vi "_Main_04_look_only.vi"() -> ()   [LabVIEW 2017]
panel:
  out "Red LED":bool
  out "Ramping":bool
  out "Heater\nEnabled":bool
  out "Heating":bool
  out "Green LED":bool
  out "unsigned 16bit integer":u16
  in  "Speed, K/min":dbl=5.0 min=0.1 max=10.0
  in  "Target, K":dbl=295.0 min=195.0 max=395.0
  in  "Ramp":bool
  out "Power LOG":cluster{dbl[], dbl[]}(graph)
  in  "Set temp":dbl=195.0 min=195.0 max=395.0
  in  "Setpoint":bool
  out "TrigTimer, s":dbl
  out "Vout, V":dbl format="%#.2g"
  out "Vin, V":dbl format="%#.5g"
  out "Temp, K":dbl
  out "Temp_sp, K":dbl
  out "Temp_gsp, K":dbl
  out "Temp LOG":cluster{dbl[], dbl[]}(graph)
  out "Bytes at Port":u32
  out "RecTry":i32
  in  "Stop Button":bool
  in  "COM port":refnum<visa-resource-name>
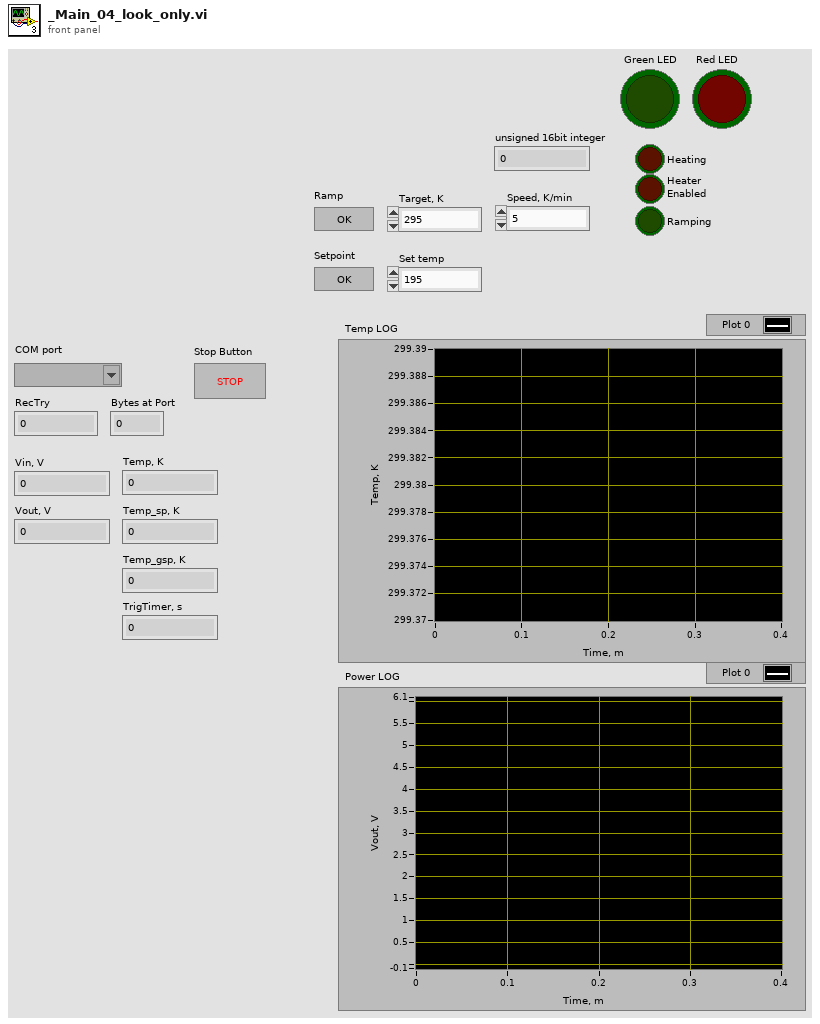
[diagram p1: front panel]
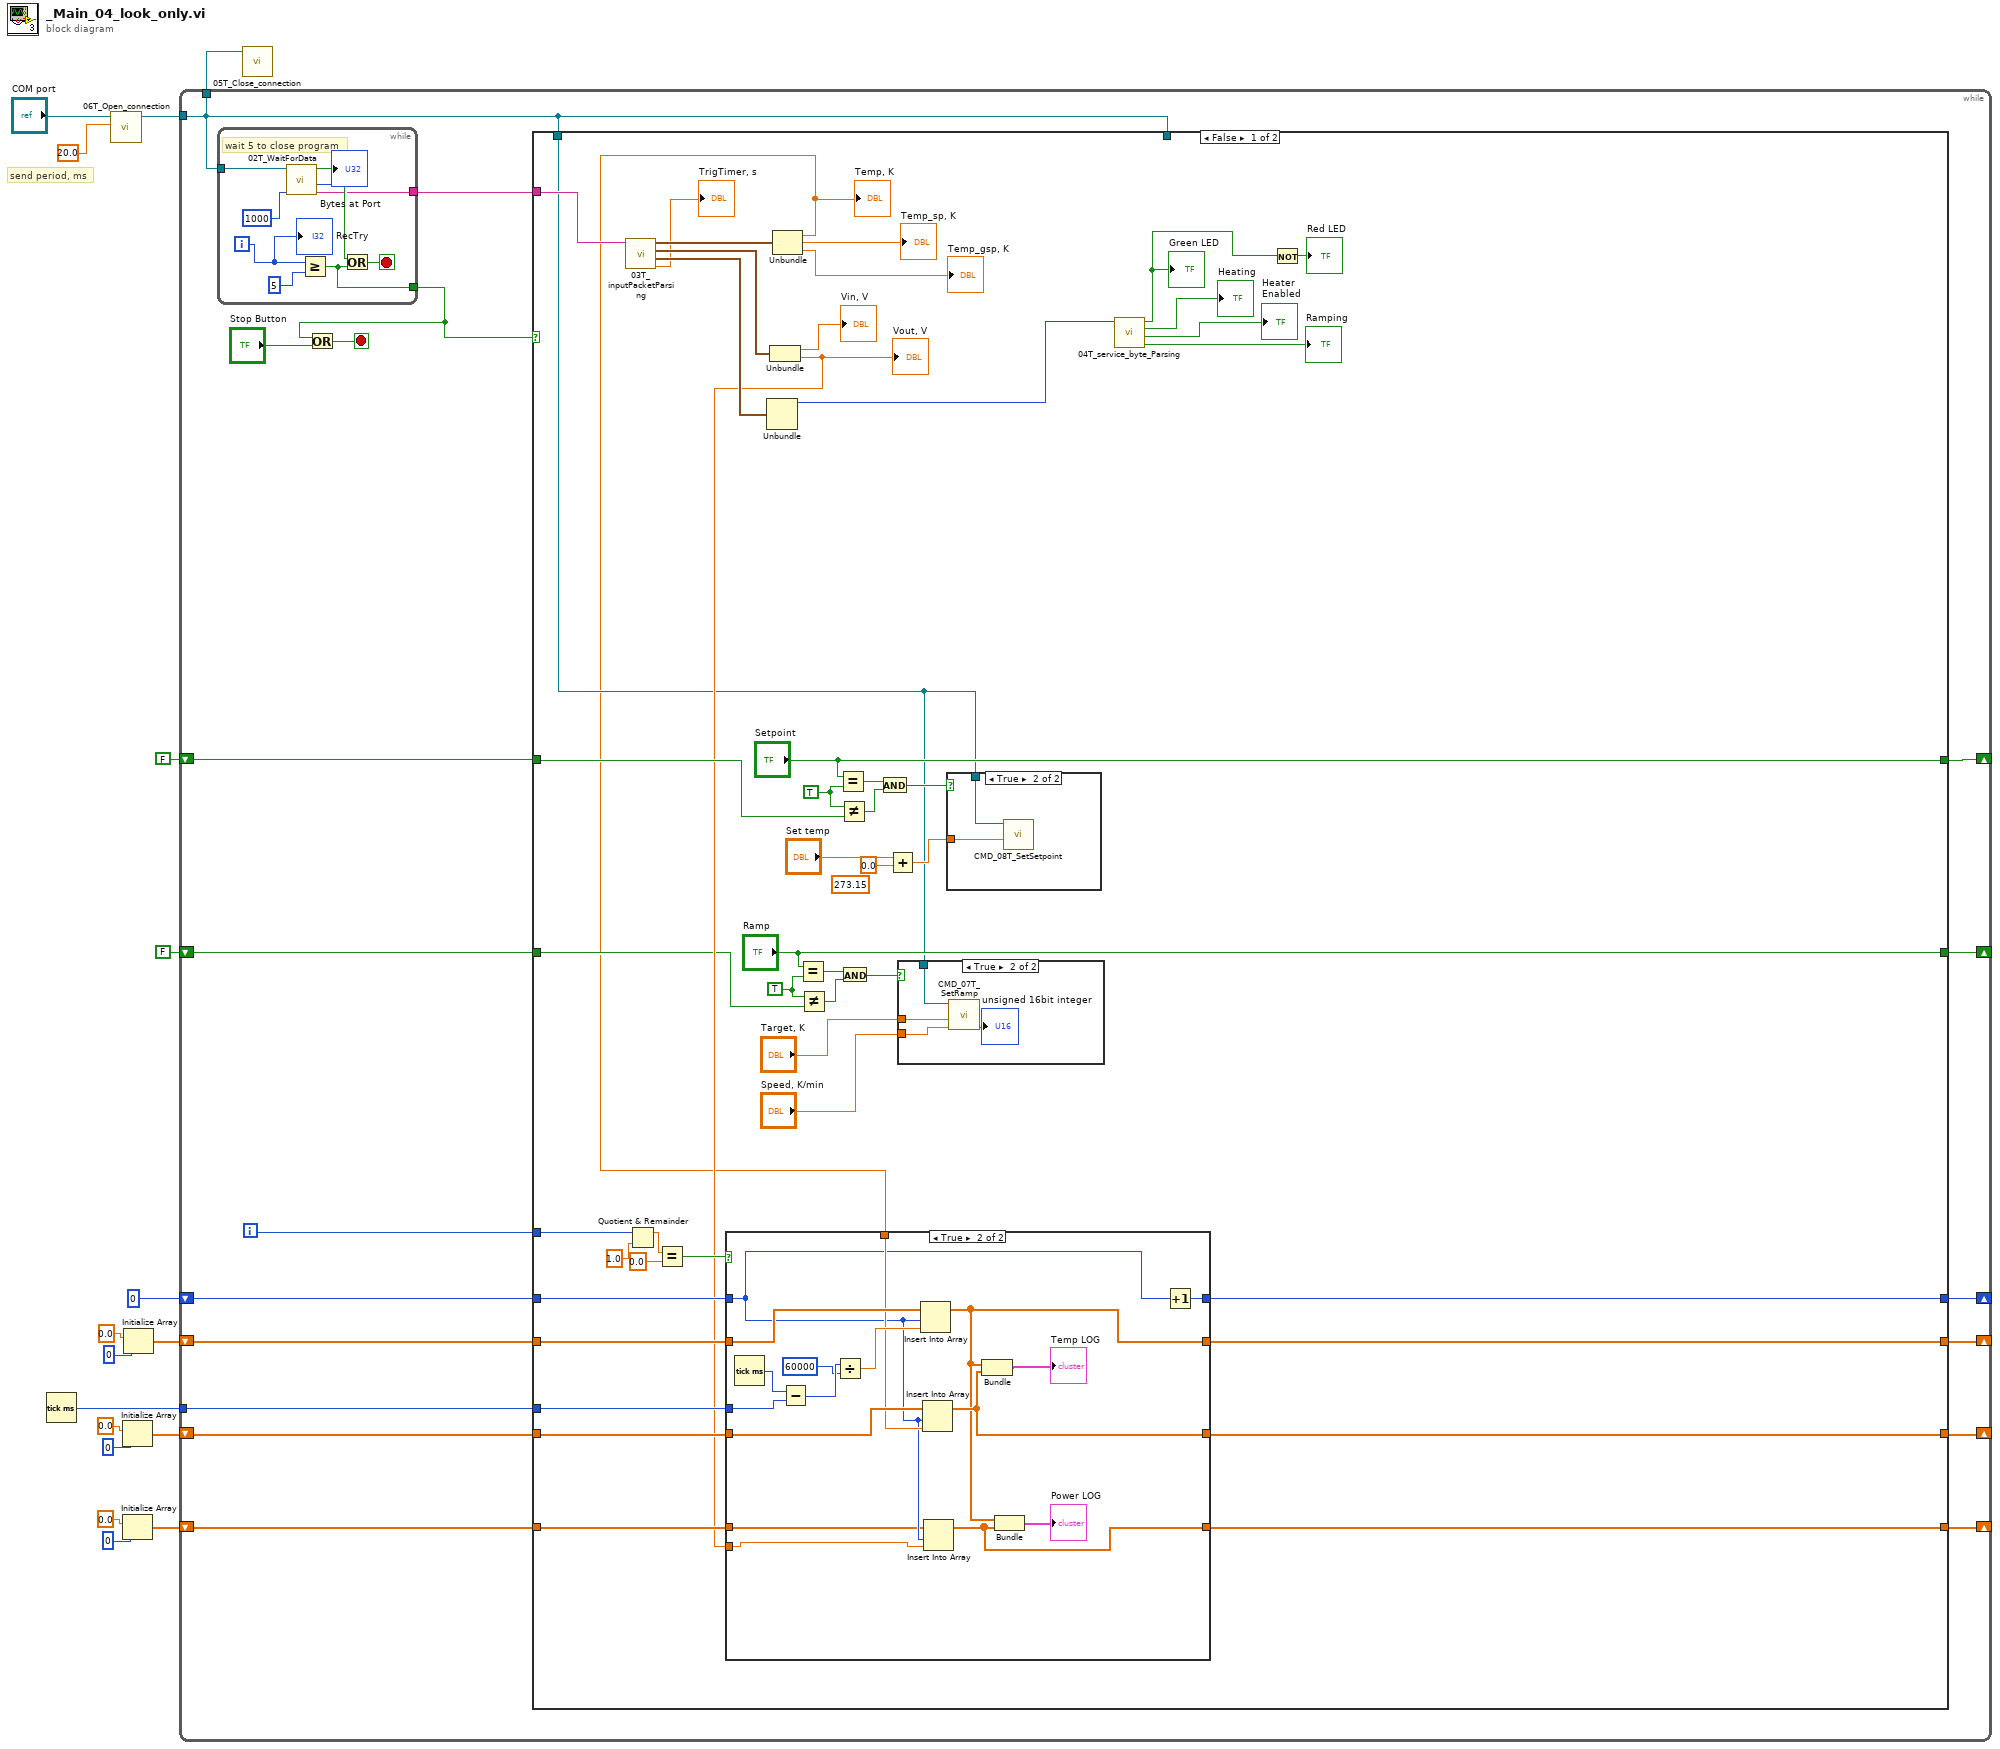
[diagram p0: block diagram]
diagram:
  # "send period, ms"
  n1 = Tick Count (ms)() -> (millisecond timer value=w13:u32)
  n2 = call "06T_Open_connection.vi"("Period, ms"=20.0, "COM port"="COM port") -> ("VISA"=w3:refnum<visa-resource-name>)  [unwired: 9 in]
  n3 = Initialize Array(0.0 ("element"), 0 ("dimension size")) -> (w10:dbl[])
  n4 = Initialize Array(0.0 ("element"), 0 ("dimension size")) -> (w6:dbl[])
  n5 = Initialize Array(0.0 ("element"), 0 ("dimension size")) -> (w14:dbl[])
  n6 = while {
    tunnel: w3 -> [w22]
    tunnel: [w22] -> w4
    shift-right: [w31] -> _
    shift-left: 0 -> [w32]
    tunnel: w13 -> [w29]
    shift-right: [w27] -> _
    shift-left: w14 -> [w30]
    shift-right: [w26] -> _
    shift-left: w10 -> [w28]
    shift-right: [w24] -> _
    shift-left: FALSE ("OK Button") -> [w23]
    shift-right: [w20] -> _
    shift-left: w6 -> [w21]
    shift-right: [w19] -> _
    shift-left: FALSE ("Ramp") -> [w18]
    i -> [w33]
    stop <- w36 stop-if-true
    n7 = while {
      tunnel: w22 -> [w118]
      tunnel: [w121] -> w35
      tunnel: [w122] -> w34
      i -> [w120]
      stop <- w124 stop-if-true
      # "wait 5 to close program"
      n8 = call "02T_WaitForData.vi"("WaitTimeoutMS"=u32 1000, "VISA"=w118) -> ("Buffer"=w122:string, "Bytes at Port"=→"Bytes at Port":u32, "Data Recived"=w123:bool)  [unwired: 7 in]
      n9 = Greater Or Equal?(x=w120, y=5) -> (x >= y?=w121:bool)
      n10 = Or(x=w123, y=w121) -> (x .or. y?=w124:bool)
      "RecTry" <- w120
    }
    n11 = Or(x=w35, y="Stop Button") -> (x .or. y?=w36:bool)
    n12 = case shown="False" w35 {
      tunnel: w34 -> [w75 _]
      tunnel: w33 -> [w81 _]
      tunnel: w22 -> [_ _]
      tunnel: w32 -> [w79 w117]
      tunnel: [w78 w117] -> w31
      tunnel: w30 -> [w68 w116]
      tunnel: w29 -> [w77 _]
      tunnel: w28 -> [w66 w115]
      tunnel: [w76 w116] -> w27
      tunnel: [w59 w115] -> w26
      tunnel: ["Setpoint" w114] -> w24
      tunnel: w23 -> [w63 w114]
      tunnel: w22 -> [w46 _]
      tunnel: w21 -> [w55 w113]
      tunnel: [w54 w113] -> w20
      tunnel: ["Ramp" w112] -> w19
      tunnel: w18 -> [w48 w112]
      frame False {
        w49 = TRUE ("y")
        (unwired) 273.15 ("y")
        w62 = TRUE ("x")
        n13 = call "03T_inputPacketParsing.vi"("string"=w75) -> ("TrigTimer, s"=→"TrigTimer, s":dbl, "Service"=w70:cluster{i32, i32, i32, i32}, "Voltage"=w71:cluster{dbl, dbl}, "Temp"=w74:cluster{dbl, dbl, dbl})  [unwired: 7 in]
        n14 = Quotient & Remainder(x=w81, y=1.0) -> (x-y*floor(x/y)=w84:dbl)  [unwired: 1 out]
        n15 = Equal?(x=w84, y=0.0) -> (x = y?=w80:bool)
        n16 = Unbundle(w70) -> (w43:i32)  [unwired: 3 out]
        n17 = Unbundle(w71) -> (→"Vin, V":dbl, w53:dbl)
        "Vout, V" <- w53
        n18 = Unbundle(w74) -> (w39:dbl, →"Temp_sp, K":dbl, →"Temp_gsp, K":dbl)
        "Temp, K" <- w39
        n19 = case shown="True" w80 {
          tunnel: w79 -> [w94 w100]
          tunnel: [w94 w107] -> w78
          tunnel: w68 -> [w92 w105]
          tunnel: w77 -> [_ w110]
          tunnel: w66 -> [w93 w104]
          tunnel: [w93 w102] -> w59
          tunnel: [w92 w98] -> w76
          tunnel: w39 -> [_ w101]
          tunnel: w55 -> [w91 w99]
          tunnel: [w91 w96] -> w54
          tunnel: w53 -> [_ w95]
          frame False {
          }
          frame True {
            n20 = Tick Count (ms)() -> (millisecond timer value=w111:u32)
            n21 = Subtract(x=w111, y=w110) -> (x-y=w109:u32)
            n22 = Divide(x=w109, y=u32 60000) -> (x/y=w106:dbl)
            n23 = Insert Into Array(array=w105, index=w100, new element=w106) -> (w98:dbl[])
            n24 = Insert Into Array(array=w104, index=w100, new element=w101) -> (w102:dbl[])
            n25 = Insert Into Array(array=w99, index=w100, new element=w95) -> (w96:dbl[])
            n26 = Bundle(w98, w102) -> (→"Temp LOG":cluster{dbl[], dbl[]})  [unwired: 1 in]
            n27 = Bundle(w98, w96) -> (→"Power LOG":cluster{dbl[], dbl[]})  [unwired: 1 in]
            n28 = Increment(x=w100) -> (x+1=w107:i32)
          }
        }
        n29 = Equal?(x="Ramp", y=w49) -> (x = y?=w52:bool)
        n30 = Not Equal?(x=w49, y=w48) -> (x != y?=w51:bool)
        n31 = Equal?(x="Setpoint", y=w62) -> (x = y?=w65:bool)
        n32 = Not Equal?(x=w62, y=w63) -> (x != y?=w61:bool)
        n33 = And(x=w52, y=w51) -> (x .and. y?=w47:bool)
        n34 = And(x=w65, y=w61) -> (x .and. y?=w60:bool)
        n35 = Add(x="Set temp", y=0.0) -> (x+y=w58:dbl)
        n36 = case shown="True" w47 {
          tunnel: w46 -> [_ w88]
          tunnel: "Target, K" -> [_ w87]
          tunnel: "Speed, K/min" -> [_ w86]
          frame False {
          }
          frame True {
            n37 = call "CMD_07T_SetRamp.vi"("Ramp speed, K/min"=w86, "Target, K"=w87, "VISA resource name"=w88) -> ("unsigned 16bit integer"=→"unsigned 16bit integer":u16)  [unwired: 7 in, 1 out]
          }
        }
        n38 = case shown="True" w60 {
          tunnel: w58 -> [_ w90]
          tunnel: w46 -> [_ w89]
          frame False {
          }
          frame True {
            n39 = call "CMD_08T_SetSetpoint.vi"("Setpoint, K"=w90, "VISA resource name"=w89) -> ()  [unwired: 9 in, 1 out]
          }
        }
        n40 = call "04T_service_byte_Parsing.vi"("Service Byte"=w43) -> ("Ramping"=→"Ramping":bool, "Heater\nEnabled"=→"Heater\nEnabled":bool, "Heating"=→"Heating":bool, "Green LED"=w37:bool)  [unwired: 7 in]
        "Green LED" <- w37
        n41 = Not(x=w37) -> (.not. x?=→"Red LED":bool)
      }
      frame True {
      }
    }
  }
  n42 = call "05T_Close_connection.vi"("VISA"=w4) -> ()  [unwired: 11 in]
